vi "angle difference.vi"(10 "angle2":dbl, 11 "angle1":dbl) -> (2 "angle diff":dbl)   [LabVIEW 2016]
panel:
  out "x-y*floor(x/y) 2":dbl
  out "x-y*floor(x/y)":dbl
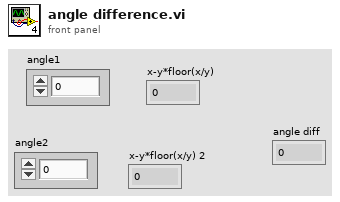
[diagram p1: front panel]
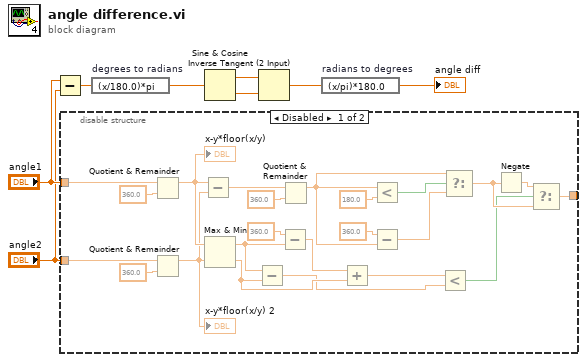
[diagram p0: block diagram]
diagram:
  n1 = Subtract(x="angle1", y="angle2") -> (x-y=w6:dbl)
  n2 = disable-structure shown="Disabled" {
    disable-tunnel: [w23 _] -> _
    disable-tunnel: "angle1" -> [w19 _]
    disable-tunnel: "angle2" -> [w18 _]
    frame Disabled {
      n3 = Quotient & Remainder(x=w19, y=360.0) -> (x-y*floor(x/y)=w10:dbl)  [unwired: 1 out]
      "x-y*floor(x/y)" <- w10
      n4 = Quotient & Remainder(x=w18, y=360.0) -> (x-y*floor(x/y)=w9:dbl)  [unwired: 1 out]
      "x-y*floor(x/y) 2" <- w9
      n5 = Subtract(x=w10, y=w9) -> (x-y=w20:dbl)
      n6 = Max & Min(x=w10, y=w9) -> (max(x,y)=w14:dbl, min(x,y)=w13:dbl)
      n7 = Subtract(x=w14, y=w13) -> (x-y=w12:dbl)
      n8 = Subtract(x=360.0, y=w14) -> (x-y=w16:dbl)
      n9 = Quotient & Remainder(x=w20, y=360.0) -> (x-y*floor(x/y)=w27:dbl)  [unwired: 1 out]
      n10 = Add(x=w16, y=w13) -> (x+y=w15:dbl)
      n11 = Less?(x=w27, y=180.0) -> (x < y?=w30:bool)
      n12 = Subtract(x=360.0, y=w27) -> (x-y=w26:dbl)
      n13 = Less?(x=w15, y=w12) -> (x < y?=w11:bool)
      n14 = Select(t=w27, s=w30, f=w26) -> (s? t:f=w21:dbl)
      n15 = Negate(x=w21) -> (-x=w22:dbl)
      n16 = Select(t=w22, s=w11, f=w21) -> (s? t:f=w23:dbl)
    }
    frame Enabled {
    }
  }
  n17 = expression code="(x/180.0)*pi" "degrees to radians"(w6) -> (w5:dbl)
  n18 = Sine & Cosine(0:w5) -> (1:w3:dbl, 2:w2:dbl)
  n19 = Inverse Tangent (2 Input)(1:w2, 2:w3) -> (0:w4:dbl)
  n20 = expression code="(x/pi)*180.0" "radians to degrees"(w4) -> (→"angle diff":dbl)
